vi "LED3 - Copy.vi"() -> ()   [LabVIEW 2024]
uses:
  <vilib>/Instr/_visa.llb/VISA Configure Serial Port (Instr).vi
panel:
  in  "LED":bool
  in  "VISA resource name":refnum<visa-resource-name>
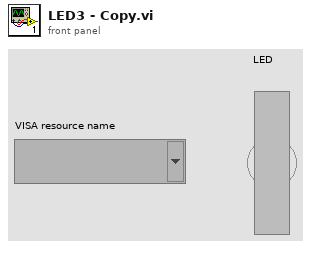
[diagram p1: front panel]
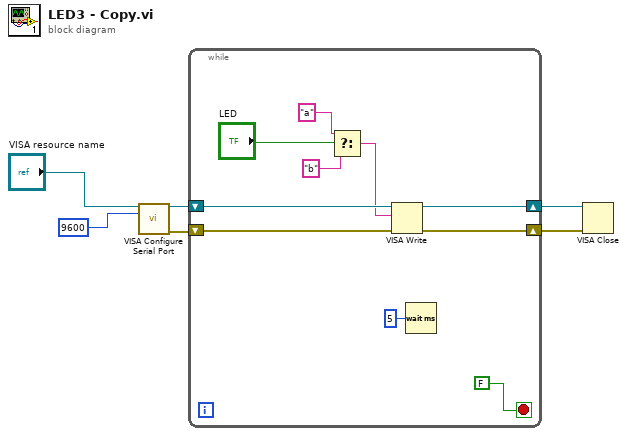
[diagram p0: block diagram]
diagram:
  n1 = call-poly "VISA Configure Serial Port"("VISA resource name"="VISA resource name", "baud rate (9600)"=u32 9600) -> ("VISA resource name out"=w6:refnum<visa-resource-name>, "error out"=w4:errorcluster)  [unwired: 12 in]
  n2 = while {
    shift-right: [w15] -> w5
    shift-left: w6 -> [w16]
    shift-right: [w13] -> w3
    shift-left: w4 -> [w14]
    stop <- FALSE stop-if-true
    n3 = Select(t="a", s="LED", f="b") -> (s? t:f=w10:string)
    n4 = VISA Write(VISA resource name=w16, write buffer=w10, error in (no error)=w14) -> (VISA resource name out=w15:refnum<visa-resource-name>, error out=w13:errorcluster)  [unwired: 1 out]
    n5 = Wait (ms)(milliseconds to wait=u32 5) -> ()  [unwired: 1 out]
  }
  n6 = VISA Close(VISA resource name=w5, error in (no error)=w3) -> ()  [unwired: 1 out]
